vi "Weighted Moving Average for Slope.vi"(11 "Slopes":dbl[](array[numeric])=[1.0, 3.0, 3.0, 3.0, 3.0, 2.0]) -> (3 "Slope":dbl)   [LabVIEW 2021, in "Time_CIF_U.lvlib"]
uses:
  Time_CIF_U.lvlib
  <vilib>/Analysis/3filter.llb/Savitzky-Golay Filter (DBL).vi
  <vilib>/Analysis/NI_AALBase.lvlib
  DataTypes/DataTypes_CIF_U.lvlib
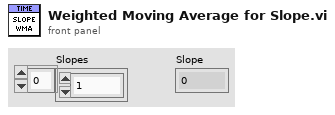
[diagram p1: front panel]
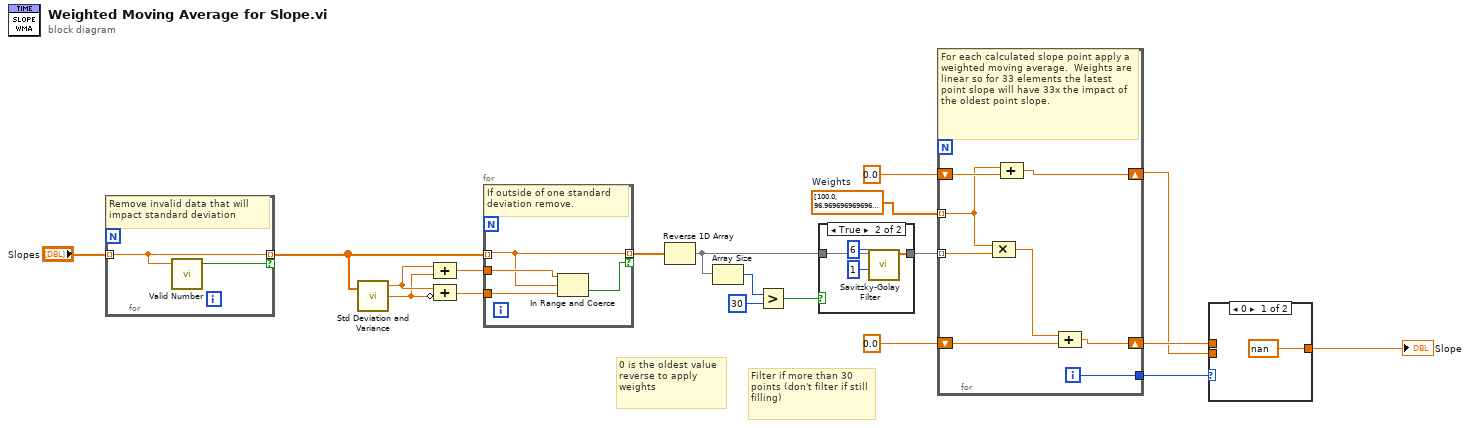
[diagram p0: block diagram]
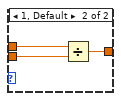
[diagram p2: hidden frame]
diagram:
  w13 = dbl[] [100.0, 96.96969696969697, 93.93939393939394, 90.9090909090909, 87.87878787878788, 84.84848484848484, 81.81818181818181, 78.78787878787878, 75.75757575757575, 72.72727272727272, 69.69696969696969, 66.66666666666666, 63.636363636363626, 60.606060606060595, 57.575757575757564, 54.54545454545453, 51.5151515151515, 48.48484848484847, 45.45454545454544, 42.42424242424241, 39.39393939393938, 36.363636363636346, 33.333333333333314, 30.303030303030283, 27.272727272727252, 24.24242424242422, 21.21212121212119, 18.18181818181816, 15.151515151515127, 12.121212121212096, 9.090909090909065, 6.060606060606035, 3.0303030303030045]  # Weights
  # "Filter if more than 30 points (don't filter if still filling)"
  # "0 is the oldest value  reverse to apply weights"
  n1 = for {
    tunnel: "Slopes" -> [w21] mode=indexing
    tunnel: [w21] -> w6 mode=indexing if=w20
    # "Remove invalid data that will impact standard deviation"
    n2 = call "Valid Number.vi"("Number"=w21) -> ("Valid"=w20:bool)  [unwired: 4 in]
  }
  n3 = call <vilib>:"Std Deviation and Variance.vi"("X"=w6) -> ("mean"=w12:dbl, "standard deviation"=w11:dbl)  [unwired: 1 in, 1 out]
  n4 = Compound Arithmetic op=ADD(w12, w11) -> (w10:dbl)
  n5 = Compound Arithmetic op=ADD(w12, invert w11) -> (w9:dbl)
  n6 = for {
    tunnel: w6 -> [w23] mode=indexing
    tunnel: w10 -> [w25]
    tunnel: w9 -> [w24]
    tunnel: [w23] -> w8 mode=indexing if=w22
    # "If outside of one standard deviation remove."
    n7 = In Range and Coerce(upper limit=w25, x=w23, lower limit=w24) -> (In Range?=w22:bool)  [unwired: 1 out]
  }
  n8 = Reverse 1D Array(array=w8) -> (reversed array=w14:dbl[])
  n9 = Array Size(array=w14) -> (size(s)=w5:i32)
  n10 = Greater?(x=w5, y=30) -> (0:w3:bool)
  n11 = case shown="True" w3 {
    tunnel: [w26 w30] -> w15
    tunnel: w14 -> [w26 w29]
    frame False {
    }
    frame True {
      n12 = call-poly <vilib>:"Savitzky-Golay Filter.vi"("polynomial order"=1, "side points"=6, "X"=w29) -> ("Filtered X"=w30:dbl[])  [unwired: 7 in, 1 out]
    }
  }
  n13 = for {
    tunnel: w15 -> [w33] mode=indexing
    shift-right: [w37] -> w19
    shift-left: 0.0 -> [w38]
    shift-right: [w35] -> w18
    shift-left: 0.0 -> [w36]
    tunnel: w13 -> [w34] mode=indexing
    tunnel: [w31] -> w1
    i -> [w31]
    # "For each calculated slope point apply a weighted moving average.  Weights are linear so for 33 elements the latest point slope will have 33x the impact of the oldest point slope."
    n14 = Compound Arithmetic op=MULTIPLY(w34, w33) -> (w32:dbl)
    n15 = Compound Arithmetic op=ADD(w34, w36) -> (w35:dbl)
    n16 = Compound Arithmetic op=ADD(w32, w38) -> (w37:dbl)
  }
  n17 = case shown="0" w1 {
    tunnel: w19 -> [_ w42]
    tunnel: w18 -> [_ w41]
    tunnel: [nan w40] -> w2
    frame 0 {
    }
    frame 1, Default {
      n18 = Divide(x=w42, y=w41) -> (x/y=w40:dbl)
    }
  }
  "Slope" <- w2
